vi "Write Update Fields Logic.vi"(8 "error in (no error)":errorcluster, 10 "Form Server Interfaces.lvlib:Update Fields Logic.lvclass":refnum<class "Update Fields Logic.lvclass">, 11 "Form Server Configuration in":refnum<class "Form Server Configuration.lvclass">) -> (0 "error out":errorcluster, 3 "Form Server Configuration out":refnum<class "Form Server Configuration.lvclass">)   [LabVIEW 2020, in "Form Server Configuration.lvlib" / "Form Server Configuration.lvclass"]
uses:
  Form Server Configuration.lvclass
  Update Fields Logic/Update Fields Logic.lvclass
  Form Server Configuration.lvclass/Form Server Configuration.ctl
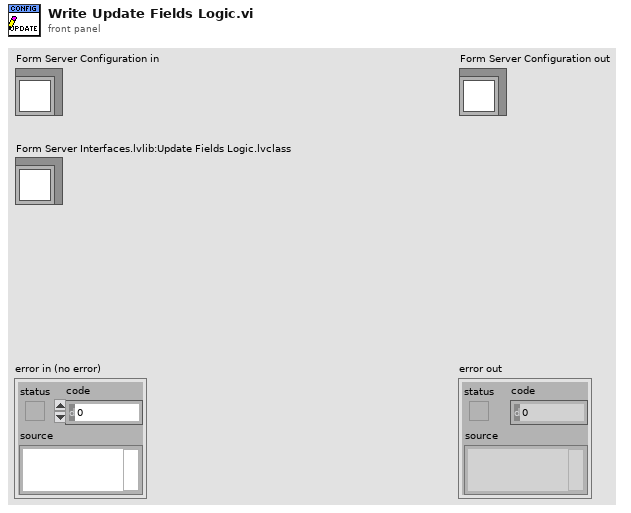
[diagram p1: front panel]
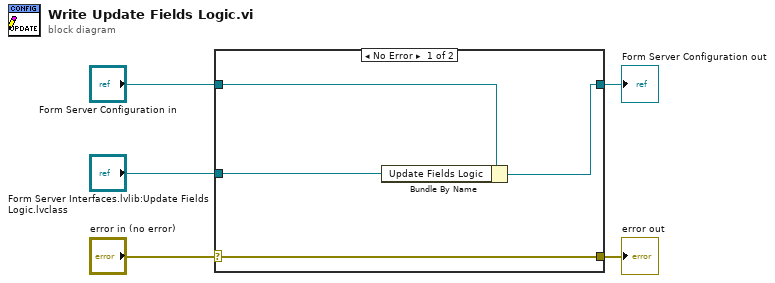
[diagram p0: block diagram]
diagram:
  n1 = case shown="No Error" "error in (no error)" {
    selector: "error in (no error)" -> [w9 w10]
    tunnel: [w9 w10] -> w4
    tunnel: [w7 w11] -> w2
    tunnel: "Form Server Configuration in" -> [w8 w11]
    tunnel: "Form Server Interfaces.lvlib:Update Fields Logic.lvclass" -> [w6 _]
    frame No Error {
      n2 = Bundle By Name(cluster=w8, "Update Fields Logic"=w6) -> (w7:refnum<class "Form Server Configuration.lvclass">)
    }
    frame Error {
    }
  }
  "error out" <- w4
  "Form Server Configuration out" <- w2
